vi "SetAnalogOutputVoltage.vi"(4 "error in (no error)":errorcluster, 5 "analog voltage value":i32, 6 "analog output number":u16, 7 "axis in":cluster{"keyHandle":u32, "nodeId":u16}={"keyHandle"=0, "nodeId"=1}) -> (0 "error out":errorcluster, 3 "axis out":cluster{"keyHandle":u32, "nodeId":u16}={"keyHandle"=0, "nodeId"=1})   [LabVIEW 2017, in "maxonEPOS.lvlib"]
doc: "<B>SetAnalogOutput</B> writes the analog value of an output to the device."
uses:
  Examples/maxonEPOS.lvlib
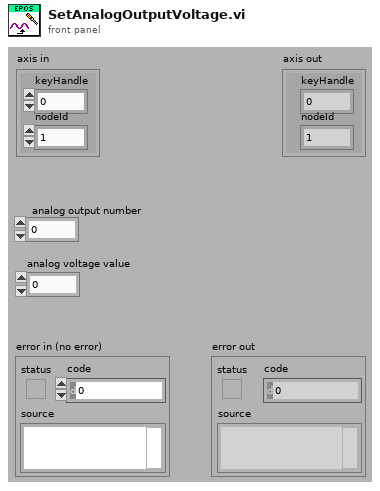
[diagram p1: front panel]
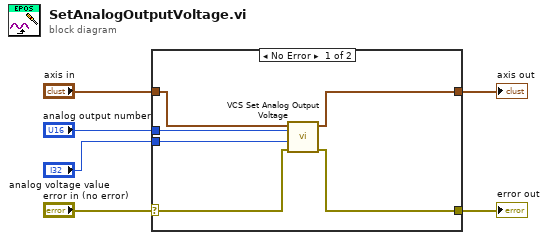
[diagram p0: block diagram]
diagram:
  n1 = case shown="No Error" "error in (no error)" {
    selector: "error in (no error)" -> [w9 w14]
    tunnel: [w10 w14] -> w5
    tunnel: [w11 w13] -> w4
    tunnel: "axis in" -> [w12 w13]
    tunnel: "analog output number" -> [w8 _]
    tunnel: "analog voltage value" -> [w7 _]
    frame No Error {
      n2 = call "VCS Set Analog Output Voltage.vi"("error in (no error)"=w9, "voltageValue"=w7, "outputNumber"=w8, "axis in"=w12) -> ("error out"=w10:errorcluster, "axis out"=w11:cluster{"keyHandle":u32, "nodeId":u16})  [unwired: 6 in]
    }
    frame Error {
    }
  }
  "error out" <- w5
  "axis out" <- w4
